vi "Start (uSMC).vi"(8 "error in":errorcluster, 9 "Index":i32, 11 "Visa Array In":refnum<visa-resource-name>[](array[refnum])) -> (0 "error out":errorcluster, 3 "Visa Array Out":refnum<visa-resource-name>[](array[refnum]))   [LabVIEW 2010, in "SignalWriterMH110203USBStepperMotor.lvclass"]
uses:
  SignalWriterMH110203USBStepperMotor.lvclass
  class_data.vi
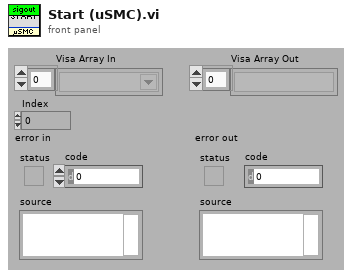
[diagram p1: front panel]
types:
  T1 = typedef "SignalWriterMH110203USBStepperMotor.lvclass/Get State Control (uSMC).ctl" = cluster{"Current Posistion":dbl, "CW/CCW":bool, "Speed":u16, "Temperature":dbl, "Power":u16, "Limit Switch 1":bool, "Limit Switch 2":bool, "After Reset":bool, "Step":u8, "Backlash":bool, "RT Error":bool, "RT State":bool, "Sync In":bool, "Sync Out":bool, "Ext Disconnect":bool, "Usb Powered":bool, "Voltage":dbl, "Working":bool, "SM Position in Encoder Units":i32, "Encoder Current Position":i32}
  T2 = typedef "SignalWriterMH110203USBStepperMotor.lvclass/Mode Control (uSMC).ctl" = cluster{"Turn Buttons Off":bool, "Reduce Current":bool, "Power Off and Make a Whole Step":bool, "Emergency Power Off":bool, "Limit Switch 1 True State":bool, "Limit Switch 2 True State":bool, "Rotary Transducer TRUE State":bool, "Swap Limit Switches":bool, "Limit Switch 1 Operation Enabled":bool, "Limit Switch 2 Operation Enabled":bool, "Rotary Transducer Operation Enabled":bool, "Rotary Transducer Operation Select":bool, "Button 1 True State":bool, "Button 2 True State":bool, "Swap Buttons":bool, "Reset Rotary Transducer Check Positions":bool, "Output Syncronization Enabled":bool, "Reset Output Sync Count":bool, "Sync Operation":bool, "Sync Count":u32, "Power":bool, "Invert Sync Polarity":bool, "Use Encoder":bool, "Invert Encoder Direction":bool, "Reset Encoder To 0":bool, "Reset SM Enc Pos to Enc Pos":bool}
  T3 = typedef "SignalWriterMH110203USBStepperMotor.lvclass/GoTo Control (uSMC).ctl" = cluster{"Step motor ID":string, "SMname":string, "Backlash":u16, "wait for input sygnal to start":bool, "use slow start/stop":bool, "units name":string, "Maximum speed":dbl, "speed":dbl, "step":u8, "point 1 ticks":i32, "point 2 ticks":i32, "point 1 units":dbl, "point 2 units":dbl, "Limit Switch standoff":dbl, "Zero Value":dbl, "Destination Position":dbl, "force backlash":bool, "power off when stop":bool, "POff delay":dbl, "positioner name":string, "R, Ohm":dbl, "I, mA":dbl, "Positioner's Type":u16, "Reset Direction":bool, "Manufacturer":string, "Model":string, "Scheme":string, "FirmwareVer":string}
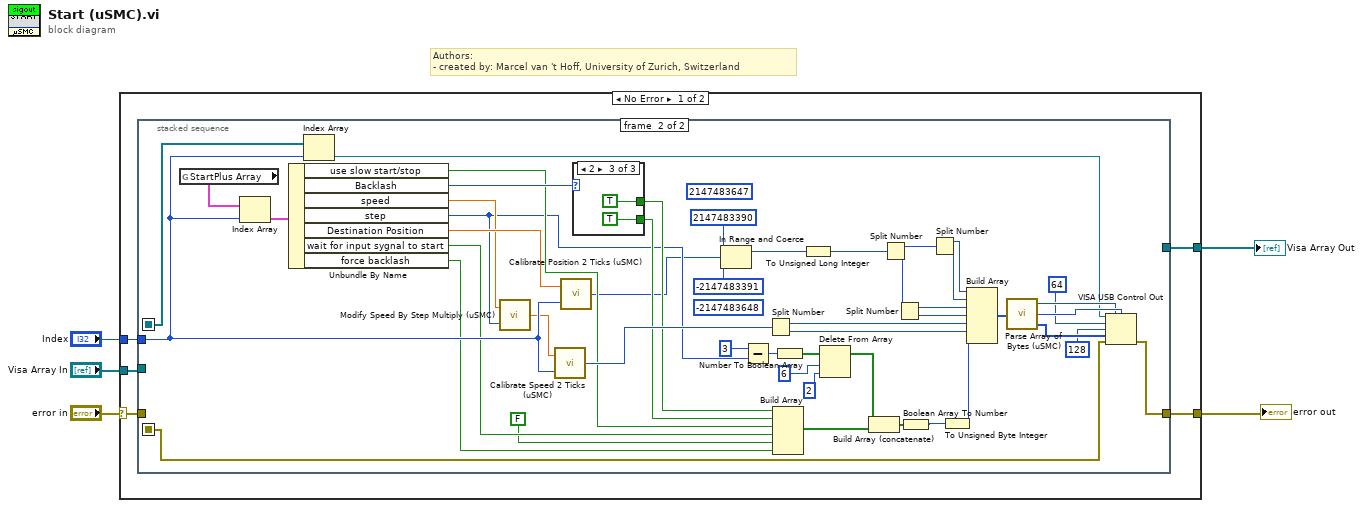
[diagram p0: block diagram]
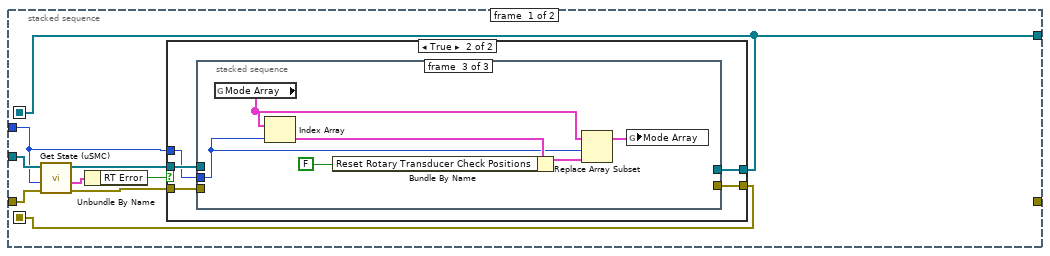
[diagram p2: hidden frame]
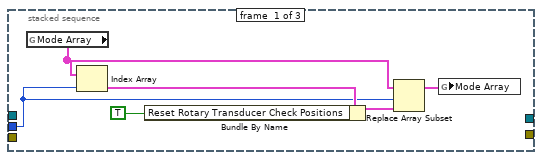
[diagram p4: hidden frame]
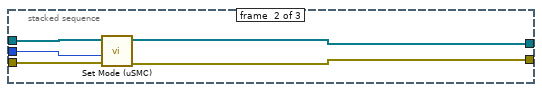
[diagram p5: hidden frame]
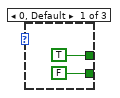
[diagram p6: hidden frame]
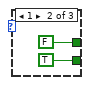
[diagram p7: hidden frame]
diagram:
  # "Authors: \n- created by: Marcel van 't Hoff, University of Zurich, Switzerland"
  n1 = case shown="No Error" "error in" {
    selector: "error in" -> [w6 w99]
    tunnel: [w10 w99] -> w5
    tunnel: "Index" -> [w9 _]
    tunnel: "Visa Array In" -> [w8 w98]
    tunnel: [w7 w98] -> w2
    frame No Error {
      n2 = stacked-sequence {
        seq-local: [w11 _] -> [_ w86]
        seq-local: [w12 _] -> [_ w60]
        tunnel: w6 -> [w14 _]
        tunnel: [_ w61] -> w10
        tunnel: w9 -> [w13 w87]
        tunnel: w8 -> [w15 _]
        tunnel: [w11 _] -> w7
        frame #0 {
          n3 = call "Get State (uSMC).vi"("error in (no error)"=w14, "SM number"=w13, "Visa array in"=w15) -> ("error out"=w19:errorcluster, "State cluster"=w17:T1, "Visa array out"=w18:refnum<visa-resource-name>[])  [unwired: 6 in]
          n4 = Unbundle By Name(w17) -> ("RT Error"=w16:bool)
          n5 = case shown="True" w16 {
            tunnel: [w20 w26] -> w12
            tunnel: [w21 w25] -> w11
            tunnel: w19 -> [w20 w24]
            tunnel: w18 -> [w21 w23]
            tunnel: w13 -> [_ w22]
            frame False {
            }
            frame True {
              n6 = stacked-sequence {
                tunnel: [_ w37 _] -> w26
                tunnel: [_ w36 _] -> w25
                tunnel: w24 -> [_ w35 _]
                tunnel: w23 -> [_ w34 _]
                tunnel: w22 -> [w29 w33 w40]
                frame #0 {
                  n7 = global read "class_data.vi" "Mode Array"() -> (w28:T2[])
                  n8 = Index Array(array=w28, index=w29) -> (element=w30:T2)
                  n9 = Bundle By Name(cluster=w30, "Reset Rotary Transducer Check Positions"=TRUE) -> (w32:T2)
                  n10 = Replace Array Subset(array=w28, new element=w32, index=w29) -> (w27:T2[])
                  n11 = global write "class_data.vi" "Mode Array"(w27) -> ()
                }
                frame #1 {
                  n12 = call "Set Mode (uSMC).vi"("error in (no error)"=w35, "Index"=w33, "Visa Array in"=w34) -> ("error out"=w37:errorcluster, "Visa Array out"=w36:refnum<visa-resource-name>[])  [unwired: 7 in]
                }
                frame #2 {
                  n13 = global read "class_data.vi" "Mode Array"() -> (w39:T2[])
                  n14 = Index Array(array=w39, index=w40) -> (element=w41:T2)
                  n15 = Bundle By Name(cluster=w41, "Reset Rotary Transducer Check Positions"=FALSE) -> (w43:T2)
                  n16 = Replace Array Subset(array=w39, new element=w43, index=w40) -> (w38:T2[])
                  n17 = global write "class_data.vi" "Mode Array"(w38) -> ()
                }
              }
            }
          }
        }
        frame #1 {
          (unwired) -2147483648 ("Abs max ticks")
          (unwired) 2147483647 ("Abs max ticks")
          n18 = global read "class_data.vi" "StartPlus Array"() -> (w91:T3[])
          n19 = Index Array(array=w91, index=w87) -> (element=w90:T3)
          n20 = Unbundle By Name(w90) -> ("use slow start/stop"=w55:bool, "Backlash"=w89:u16, "speed"=w49:dbl, "step"=w48:u8, "Destination Position"=w88:dbl, "wait for input sygnal to start"=w54:bool, "force backlash"=w53:bool)
          n21 = Index Array(array=w86, index=w87) -> (element=w52:refnum<visa-resource-name>)
          n22 = call "Modify Speed By Step Multiply (uSMC).vi"("Step"=w48, "Speed"=w49) -> ("speed"=w50:dbl)
          n23 = call "Calibrate Speed 2 Ticks (uSMC).vi"("Index"=w87, "speed value (units)"=w50) -> ("speed ticks"=w59:u16)
          n24 = call "Calibrate Position 2 Ticks (uSMC).vi"("array index"=w87, "value"=w88) -> ("value ticks"=w47:i32)
          n25 = case shown="2" w89 {
            tunnel: [TRUE FALSE TRUE] -> w57
            tunnel: [FALSE TRUE TRUE] -> w56
            frame 0, Default {
            }
            frame 1 {
            }
            frame 2 {
            }
          }
          n26 = In Range and Coerce(upper limit=2147483390 ("Abs max ticks"), x=w47, lower limit=-2147483391 ("Abs min ticks")) -> (coerced(x)=w46:i32)  [unwired: 1 out]
          n27 = Subtract(x=u8 3, y=w48) -> (x-y=w63:u8)
          n28 = Split Number(x=w59) -> (hi(x)=w71:u8, lo(x)=w72:u8)
          n29 = Build Array(w57, w56, w55, w54, FALSE, w53) -> (w58:bool[])
          n30 = Number To Boolean Array(number=w63) -> (Boolean array=w66:bool[])
          n31 = To Unsigned Long Integer(number=w46) -> (unsigned 32bit integer=w70:u32)
          n32 = Delete From Array(array=w66, length=6, index=2) -> (array with subset deleted=w67:bool[])  [unwired: 1 out]
          n33 = Build Array (concatenate)(w67, w58) -> (w65:bool[])
          n34 = Split Number(x=w70) -> (hi(x)=w77:u16, lo(x)=w76:u16)
          n35 = Split Number(x=w76) -> (hi(x)=w80:u8, lo(x)=w81:u8)
          n36 = Boolean Array To Number(Boolean array=w65) -> (number=w64:u32)
          n37 = Split Number(x=w77) -> (hi(x)=w78:u8, lo(x)=w79:u8)
          n38 = To Unsigned Byte Integer(number=w64) -> (unsigned 8bit integer=w73:u8)
          n39 = Build Array(w78, w79, w80, w81, w71, w72, w73) -> (w85:u8[])
          n40 = call "Parse Array of Bytes (uSMC).vi"("byte array"=w85) -> ("first 2 bytes"=w83:u16, "second 2 bytes"=w84:u16, "array buffer"=w82:u8[])
          n41 = VISA USB Control Out(0:w52, 1:w83, 2:w84, 5:i16 64 ("request type"), 7:i16 128 ("request type"), 9:w82, 11:w60) -> (15:w61:errorcluster)  [unwired: 1 out]
        }
      }
    }
    frame Error {
    }
  }
  "error out" <- w5
  "Visa Array Out" <- w2
